vi "SLL DE AO Safe Values.vi"(8 "error in (no error)":errorcluster) -> (0 "error out":errorcluster, 2 "AO Safe Values":dbl[](array[numeric]) format="%.2f", 3 "AO Channels (Enum)":T1[](array[typedef]))   [LabVIEW 2013]
doc: "Copyright © 2005, Soliton Technologies.\nAll rights reserved."
uses:
  Controls/SLL DE List of Analog Outputs.ctl
  Controls/SLL DE AO Min Max Range Checking Options.ctl
  Controls/SLL DE AO Safe Value Global Options.ctl
panel:
  in  "List of Analog Outputs":T1
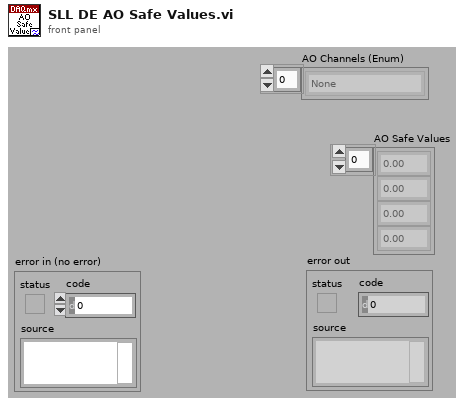
[diagram p1: front panel]
types:
  T1 = typedef "SLL DE List of Analog Outputs.ctl" = enum16{"None"}
  T2 = typedef "SLL DE AO Safe Value Global Options.ctl" = enum16{"Read", "Write"}
  T3 = typedef "SLL DE AO Min Max Range Checking Options.ctl" = enum16{"Initalize Channel Range", "Check Single AO Channel", "Check Multiple AO Channels"}
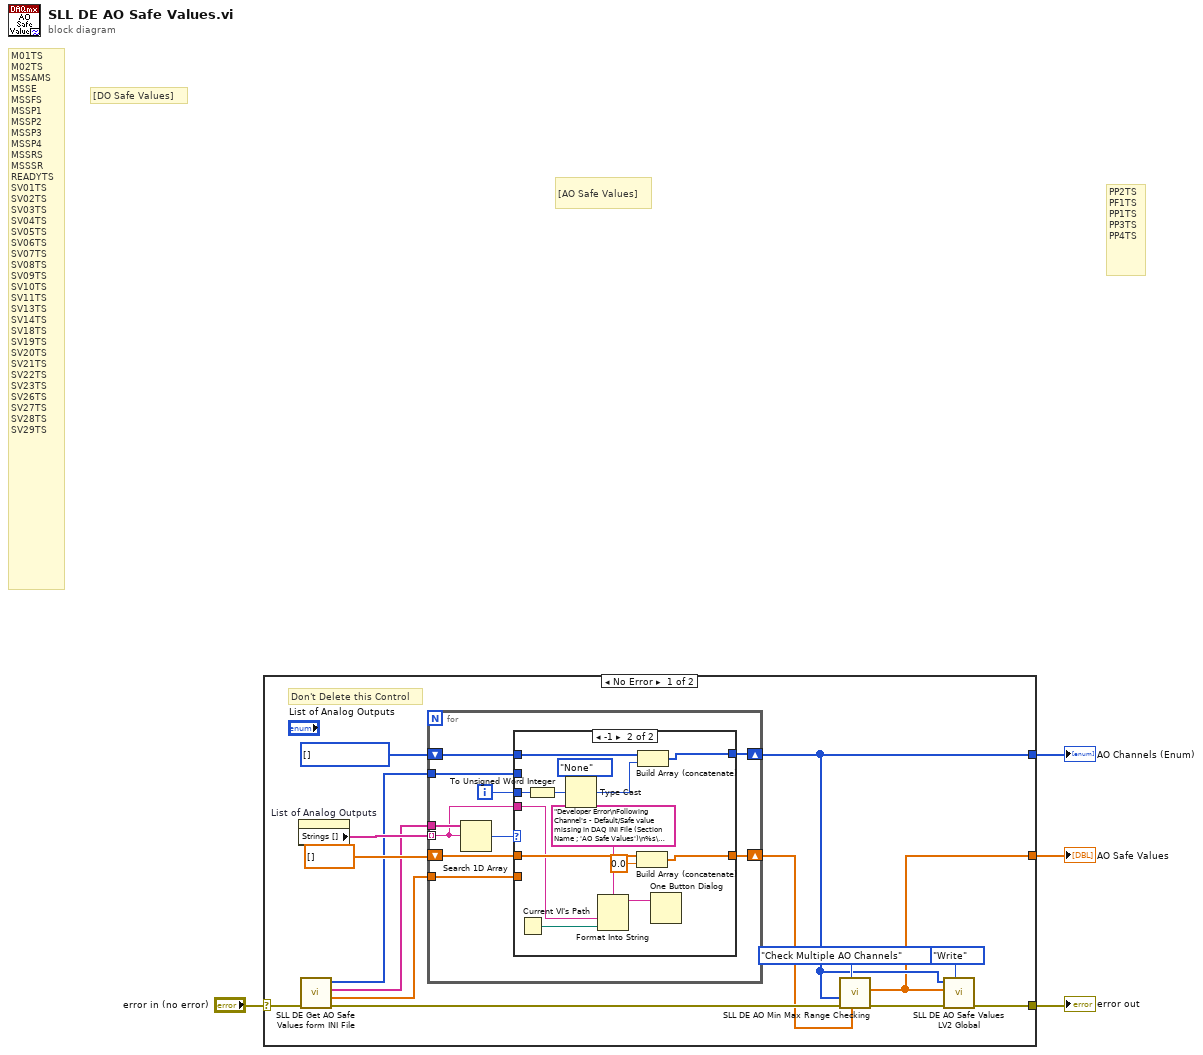
[diagram p0: block diagram]
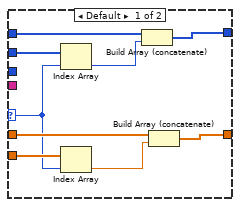
[diagram p2: hidden frame]
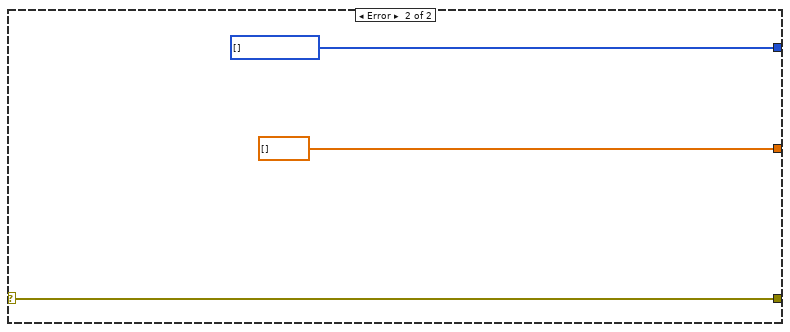
[diagram p3: hidden frame]
diagram:
  # "[DO Safe Values]"
  # "PP2TS\nPF1TS\nPP1TS\nPP3TS\nPP4TS"
  # "[AO Safe Values]"
  # "M01TS\nM02TS\nMSSAMS\nMSSE\nMSSFS\nMSSP1\nMSSP2\nMSSP3\nMSSP4\nMSSRS\nMSSSR\nREADYTS\nSV01TS\nSV02TS\nSV03TS\nSV04TS\nSV05TS\nSV06TS\nSV07TS\nSV08TS\nSV09TS\nSV10TS\nSV11TS\nSV13TS\nSV14TS\nSV18TS\nSV19TS\nSV20TS\nSV21TS\nSV22TS\nSV23TS\nSV26TS\nSV27TS\nSV28TS\nSV29TS"
  n1 = case shown="No Error" "error in (no error)" {
    selector: "error in (no error)" -> [w12 w54]
    tunnel: [w14 w54] -> w3
    tunnel: [w5 dbl[] [] ("Key Values")] -> w2
    tunnel: [w13 w52] -> w1
    frame No Error {
      w7 = T1[] [] items=["None"]
      # "Don't Delete this Control"
      n2 = property on="List of Analog Outputs" class="Enum (strict)"() -> ("Strings []"=w19:string[])  [unwired: 2 in, 2 out]
      n3 = call "SLL DE Get AO Safe Values form INI File.vi"("error in (no error)"=w12) -> ("error out"=w11:errorcluster, "AO Safe Values"=w9:dbl[], "AO Channel Names (String)"=w10:string[], "AO Channels (Enum)"=w8:T1[])  [unwired: 7 in]
      n4 = for {
        tunnel: w10 -> [w29]
        tunnel: w19 -> [w24] mode=indexing
        tunnel: w9 -> [w27]
        shift-right: [w26] -> w6
        shift-left: dbl[] [] -> [w25]
        tunnel: w8 -> [w23]
        shift-right: [w22] -> w13
        shift-left: w7 -> [w21]
        i -> [w20]
        n5 = Search 1D Array(1D array=w29, element=w24) -> (index of element=w28:i32)  [unwired: 1 in]
        n6 = case shown="-1" w28 {
          selector: w28 -> [w33 _]
          tunnel: w27 -> [w38 _]
          tunnel: [w37 w49] -> w26
          tunnel: w25 -> [w35 w51]
          tunnel: w24 -> [_ w45]
          tunnel: w23 -> [w34 _]
          tunnel: [w31 w43] -> w22
          tunnel: w21 -> [w30 w44]
          tunnel: w20 -> [_ w42]
          frame Default {
            n7 = Index Array(array=w34, index=w33) -> (element=w32:T1)
            n8 = Index Array(array=w38, index=w33) -> (element=w36:dbl)
            n9 = Build Array (concatenate)(w30, w32) -> (w31:T1[])
            n10 = Build Array (concatenate)(w35, w36) -> (w37:dbl[])
          }
          frame -1 {
            n11 = Current VI's Path() -> (path=w48:path)
            n12 = To Unsigned Word Integer(number=w42) -> (unsigned 16bit integer=w41:u16)
            n13 = Type Cast(type=SLL_DE_List_of_Analog_Outputs."None" ("List of Analog Outputs"), x=w41) -> (*(type *) &x=w40:T1)
            n14 = Format Into String(format string="Developer Error\nFollowing Channel's - Default/Safe value missing in DAQ INI File (Section Name ; 'AO Safe Values')\n%s\n%s" ("message"), w45, w48) -> (resulting string=w47:string)  [unwired: 2 in, 1 out]
            n15 = Build Array (concatenate)(w51, 0.0 ("element")) -> (w49:dbl[])
            n16 = Build Array (concatenate)(w44, w40) -> (w43:T1[])
            n17 = One Button Dialog(message=w47) -> ()  [unwired: 1 in, 1 out]
          }
        }
      }
      n18 = call "SLL DE AO Min Max Range Checking.vi"("AO Values In"=w6, "Option"=SLL_DE_AO_Min_Max_Range_Checking_Options."Check Multiple AO Channels", "error in (no error)"=w11, "AO Channels Name"=w13) -> ("error out"=w17:errorcluster, "AO Values Out"=w5:dbl[])  [unwired: 5 in, 1 out]
      n19 = call "SLL DE AO Safe Values LV2 Global.vi"("Cases"=SLL_DE_AO_Safe_Value_Global_Options."Write", "error in (no error)"=w17, "Value In"=w5, "Elements In"=w13) -> ("error out"=w14:errorcluster)  [unwired: 5 in, 2 out]
    }
    frame Error {
      w52 = T1[] [] items=["None"]
    }
  }
  "error out" <- w3
  "AO Safe Values" <- w2
  "AO Channels (Enum)" <- w1
